vi "Set Initialization Data - Servo_Emulator.vi"(8 "error in":errorcluster, 11 "Device Manager in":refnum<class "Device Manager.lvclass">) -> (0 "error out":errorcluster, 3 "Device Manager out":refnum<class "Device Manager.lvclass">)   [LabVIEW 2017, in "Device Manager.lvclass"]
doc: "In this VI you can set the initialization data of a statically-linked subWorker."
uses:
  Device Manager.lvclass
  Servo Motor Emulator/Initialization Data.ctl
  Servo Motor Emulator/Response Cases.ctl
  <vilib>/addons/_Workers/Library/Case Label.ctl
  Device Manager.lvclass/Device Manager.ctl
  Servo Motor Emulator/Servo Motor Emulator.lvclass
  C:/Program Files (x86)/National Instruments/LabVIEW 2017/vi.lib/addons/_Workers/Library/Classes/Worker/Worker.lvclass
  <vilib>/addons/_Workers/Library/Workers.lvlib
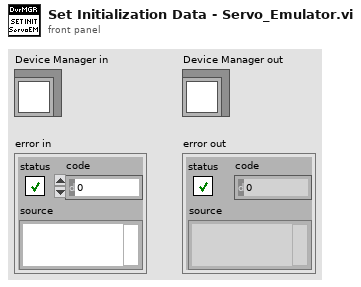
[diagram p1: front panel]
types:
  T1 = typedef "Servo Motor Emulator.lvclass/Initialization Data.ctl" = cluster{"Response Cases":T2}
  T2 = typedef "Servo Motor Emulator.lvclass/Response Cases.ctl" = cluster{"Report Temperature":T3, "Report Humidity":T3}
  T3 = typedef "Workers.lvlib/Case Label.ctl" = string
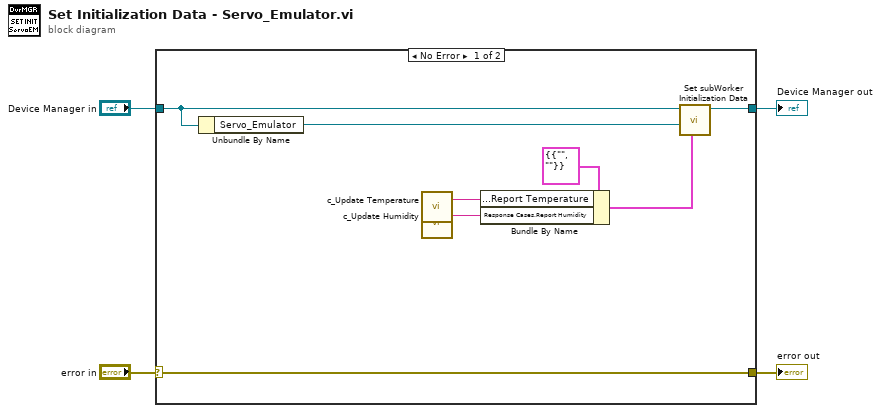
[diagram p0: block diagram]
diagram:
  n1 = case shown="No Error" "error in" {
    selector: "error in" -> [w12 w14]
    tunnel: [w12 w14] -> w3
    tunnel: [w10 w13] -> w2
    tunnel: "Device Manager in" -> [w9 w13]
    frame No Error {
      n2 = Unbundle By Name(w9) -> ("Servo_Emulator"=w11:refnum<class "Servo Motor Emulator.lvclass">)
      n3 = call "c_Update Temperature.vi"() -> ("Case Label"=w6:T3)  [unwired: 1 in]
      n4 = call "c_Update Humidity.vi"() -> ("Case Label"=w5:T3)  [unwired: 1 in]
      n5 = Bundle By Name(cluster=T1 {"Response Cases"={"Report Temperature"="", "Report Humidity"=""}} ("Initialization Data"), "Response Cases.Report Temperature"=w6, "Response Cases.Report Humidity"=w5) -> (w7:T1)
      n6 = call-dynamic "Set subWorker Initialization Data.vi"("Initialization Data"=w7, "subWorker"=w11, "Worker"=w9) -> ("Worker out"=w10:refnum<class "Device Manager.lvclass">)  [unwired: 8 in]
    }
    frame Error {
    }
  }
  "error out" <- w3
  "Device Manager out" <- w2
